vi "SetGeometry.vi"(8 "error in (no error)":errorcluster, 10 "Geometry":refnum<vi>, 11 "Object in":refnum<class "3D Object.lvclass">) -> (0 "error out":errorcluster, 3 "Object out":refnum<class "3D Object.lvclass">)   [LabVIEW 2015, in "3D Object.lvclass"]
uses:
  3D Object.lvclass
  3D Object.lvclass/3D Object.ctl
  <vilib>/picture/3D Picture Control/Object/Create Object (name).vi
  <vilib>/picture/3D Picture Control/NI_3D Picture Control.lvlib
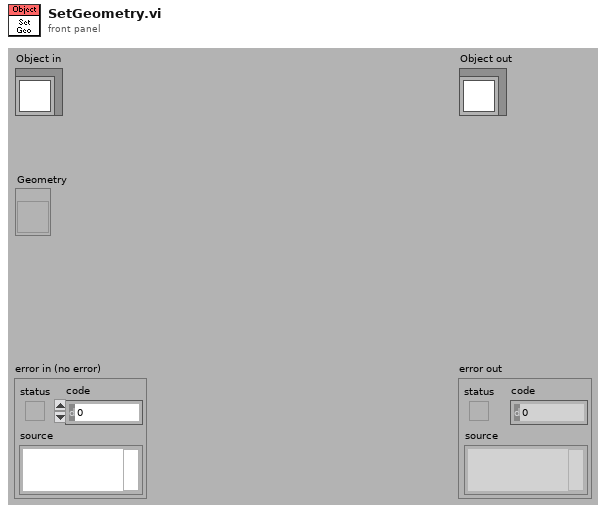
[diagram p1: front panel]
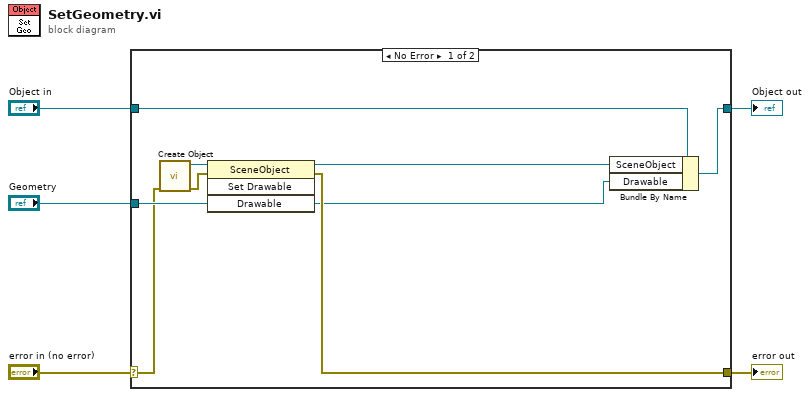
[diagram p0: block diagram]
diagram:
  n1 = case shown="No Error" "error in (no error)" {
    selector: "error in (no error)" -> [w9 w16]
    tunnel: [w7 w16] -> w4
    tunnel: [w13 w15] -> w2
    tunnel: "Object in" -> [w14 w15]
    tunnel: "Geometry" -> [w10 _]
    frame No Error {
      n2 = call-poly <vilib>:"Create Object.vi"("error in (no error)"=w9) -> ("error out"=w11:errorcluster, "Scene:New Object"=w12:refnum<vi>)  [unwired: 9 in]
      n3 = invoke class="SceneObject" method="Set Drawable"(reference=w12, error in=w11, "Drawable"=w10) -> (reference out=w8:refnum<vi>, error out=w7:errorcluster, "Drawable"=w6:refnum<vi>)  [unwired: 1 in, 1 out]
      n4 = Bundle By Name(cluster=w14, "SceneObject"=w8, "Drawable"=w6) -> (w13:refnum<class "3D Object.lvclass">)
    }
    frame Error {
    }
  }
  "error out" <- w4
  "Object out" <- w2
